vi "E3643A Initial Setup.vi"(6 "Level (0.0 Volts)":dbl, 7 "Combo Box":string(combo), 8 "Error In":errorcluster, 9 "Output ENA?":bool, 10 "Init?":bool, 11 "VISA resource In":refnum<visa-resource-name>) -> (0 "Error Out":errorcluster, 3 "VISA resource Out":refnum<visa-resource-name>)   [LabVIEW 2017]
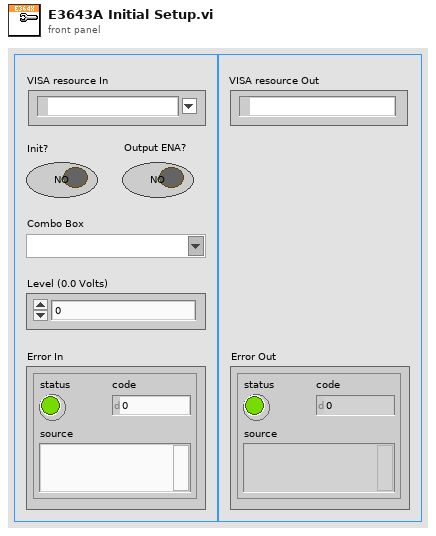
[diagram p1: front panel]
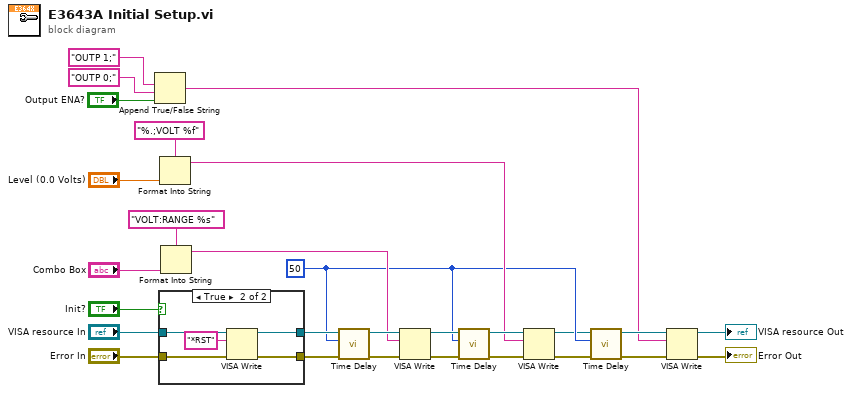
[diagram p0: block diagram]
diagram:
  w9 = u32 50 ("Delay(ms)")
  n1 = Append True/False String(1:"Output ENA?", 2:"OUTP 0;" ("true string"), 3:"OUTP 1;" ("true string")) -> (0:w1:string)  [unwired: 1 in]
  n2 = case shown="True" "Init?" {
    tunnel: "VISA resource In" -> [w27 w32]
    tunnel: "Error In" -> [w26 w30]
    tunnel: [w26 w29] -> w14
    tunnel: [w27 w28] -> w22
    frame False {
    }
    frame True {
      n3 = VISA Write(VISA resource name=w32, write buffer="*RST", error in (no error)=w30) -> (VISA resource name out=w28:refnum<visa-resource-name>, error out=w29:errorcluster)  [unwired: 1 out]
    }
  }
  n4 = Format Into String(format string="%.;VOLT %f", "Level (0.0 Volts)") -> (resulting string=w11:string)  [unwired: 2 in, 1 out]
  n5 = Format Into String(format string="VOLT:RANGE %s", "Combo Box") -> (resulting string=w19:string)  [unwired: 2 in, 1 out]
  n6 = call "Time Delay.vi"("Error In"=w14, "Delay(ms)"=w9) -> ("Error Out"=w15:errorcluster)  [unwired: 9 in]
  n7 = VISA Write(VISA resource name=w22, write buffer=w19, error in (no error)=w15) -> (VISA resource name out=w18:refnum<visa-resource-name>, error out=w16:errorcluster)  [unwired: 1 out]
  n8 = call "Time Delay.vi"("Error In"=w16, "Delay(ms)"=w9) -> ("Error Out"=w17:errorcluster)  [unwired: 9 in]
  n9 = VISA Write(VISA resource name=w18, write buffer=w11, error in (no error)=w17) -> (VISA resource name out=w5:refnum<visa-resource-name>, error out=w10:errorcluster)  [unwired: 1 out]
  n10 = call "Time Delay.vi"("Error In"=w10, "Delay(ms)"=w9) -> ("Error Out"=w6:errorcluster)  [unwired: 9 in]
  n11 = VISA Write(VISA resource name=w5, write buffer=w1, error in (no error)=w6) -> (VISA resource name out=→"VISA resource Out":refnum<visa-resource-name>, error out=→"Error Out":errorcluster)  [unwired: 1 out]
